vi "Write configuration.vi"(8 "error in":errorcluster, 10 "TBM configuration in":refnum<class "NISE_CEF_serializable configuration.lvclass">, 11 "Profibus Module editor node in":refnum<class "Profibus Module editor node.lvclass">) -> (0 "error out":errorcluster, 3 "Profibus Module editor node out":refnum<class "Profibus Module editor node.lvclass">)   [LabVIEW 2013, in "Profibus Module editor node.lvclass"]
uses:
  Profibus Module editor node.lvclass
  configuration/Profibus Module configuration.lvclass
  <vilib>/NI/Configuration Framework/serializable configuration/NISE_CEF_serializable configuration.lvclass
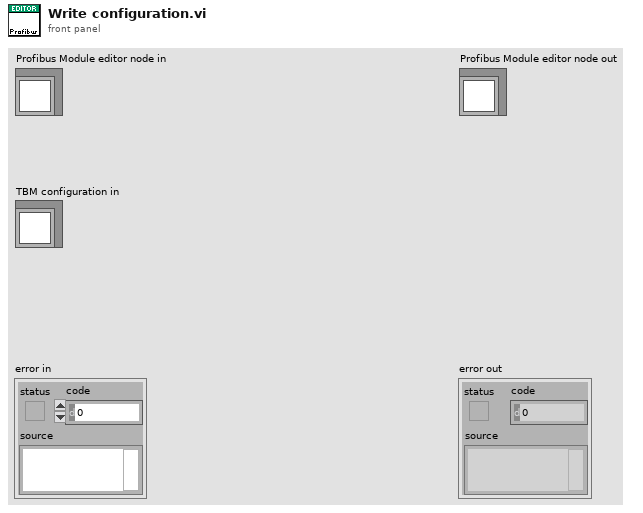
[diagram p1: front panel]
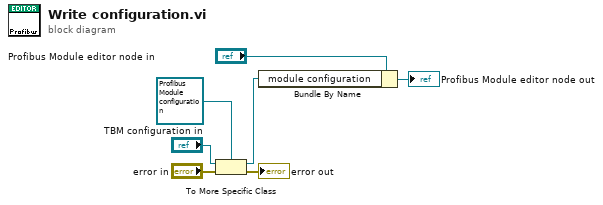
[diagram p0: block diagram]
diagram:
  n1 = To More Specific Class(target class=refnum<class "Profibus Module configuration.lvclass"> refnum ("module configuration"), reference="TBM configuration in", error in="error in") -> (specific class reference=w1:refnum<class "Profibus Module configuration.lvclass">, error out=→"error out":errorcluster)
  n2 = Bundle By Name(cluster="Profibus Module editor node in", "module configuration"=w1) -> (→"Profibus Module editor node out":refnum<class "Profibus Module editor node.lvclass">)
